vi "EmergencyManifoldTemperature (1).vi"(1 "Numeric":dbl) -> (0 "Boolean":bool)   [LabVIEW 2017]
uses:
  EmergencyGLOBAL.vi
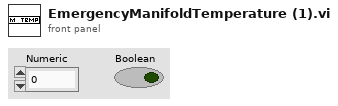
[diagram p1: front panel]
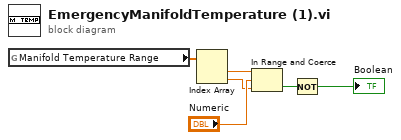
[diagram p0: block diagram]
diagram:
  n1 = global read "EmergencyGLOBAL.vi" "Manifold Temperature Range"() -> (w2:dbl[])
  n2 = Index Array(array=w2) -> (element #1=w4:dbl, element #2=w3:dbl)  [unwired: 2 in]
  n3 = In Range and Coerce(upper limit=w4, x="Numeric", lower limit=w3) -> (In Range?=w5:bool)  [unwired: 1 out]
  n4 = Not(x=w5) -> (.not. x?=→"Boolean":bool)
